vi "Micro-PL Drive Calibration v10.5.1.vi"() -> ()   [LabVIEW 2010]
uses:
  <vilib>/Utility/miscctls.llb/LVPointTypeDef.ctl
  subvi/ESA-C/TypeDefs/ESA-C Connection Settings.ctl
  <vilib>/Utility/file.llb/Write To Spreadsheet File (DBL).vi
panel:
  in  "Snapshot Folder":path=path "C:/Users/WET-KORR/Desktop/Screenshots"
  in  "Camera Name":string="HD USB Camera"
  in  "GPIB-Port":u8=4 max=150 step=1
  in  "Start":bool
  out "Voltages":ext[][](array[numeric])
  out "Current Voltage":ext caption="Current (V)" format="%.1f"
  in  "Axis":u16(ring)=1 items=["X"=1, "Y"=2, "Z"=3]
  out "Progress":u8(slide) max=10 scale=0.0..100.0
  in  "Exit":bool
  in  "Voltage Step":dbl=1.0 caption="Step (V)" min=0.1 max=30.0 step=0.1
  # "Drive Calibration"
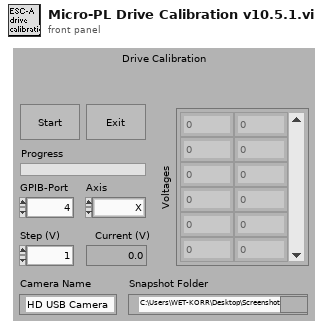
[diagram p1: front panel]
types:
  T1 = typedef "LVPointTypeDef.ctl" = cluster{"Horizontal":i16, "Vertical":i16}
  T2 = typedef "ESA-C Connection Settings.ctl" = cluster{"Objective GPIB-Port":i32, "Stage GPIB-Port":i32, "Drive Selector":u16, "Drive Velocity (V/s)":dbl}
  T3 = typedef "ESA-C Current Values.ctl" = cluster{"Voltages":cluster{"Drive X Voltage":dbl, "Drive Y Voltage":dbl, "Drive Z Voltage":dbl}, "Position":cluster{"Drive X Position":dbl, "Drive Y Position":dbl, "Drive Z Position":dbl}}
  T4 = cluster{"Drive X Voltage":dbl, "Drive Y Voltage":dbl, "Drive Z Voltage":dbl}
  T5 = enum32{"invalid app kind", "Development System", "Run Time System", "Student Edition", "Embedded LabVIEW", "Evaluation", "Custom"}
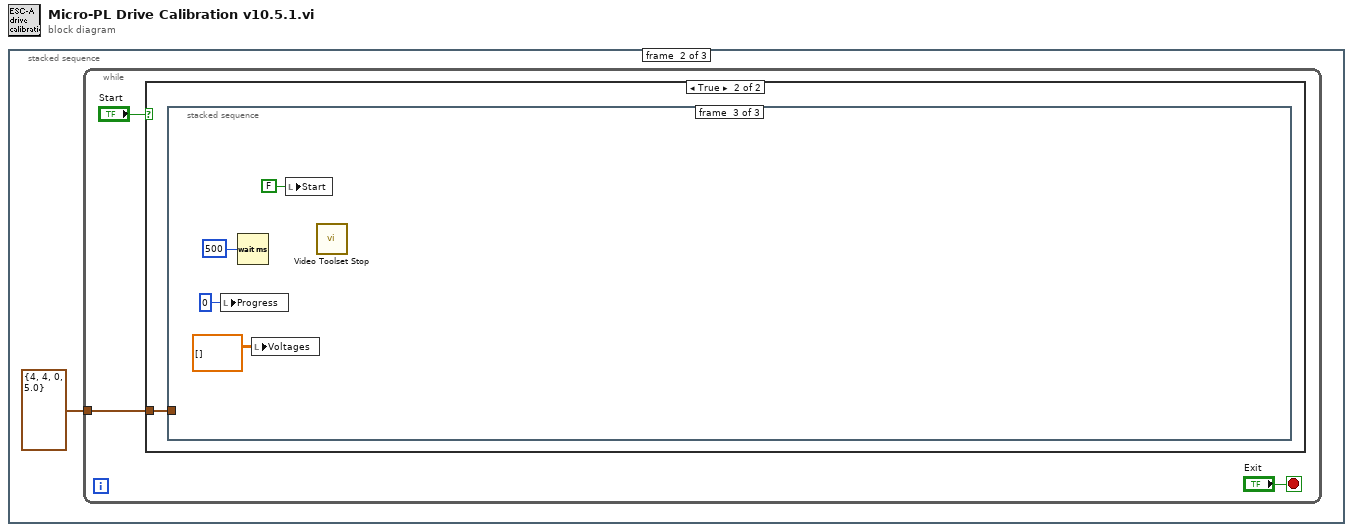
[diagram p0: block diagram]
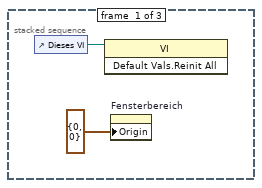
[diagram p2: hidden frame]
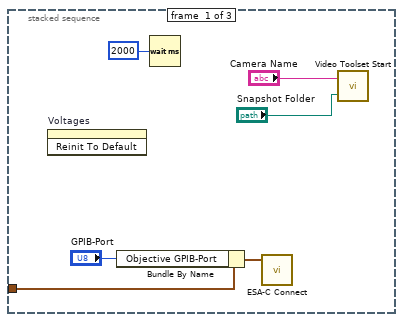
[diagram p4: hidden frame]
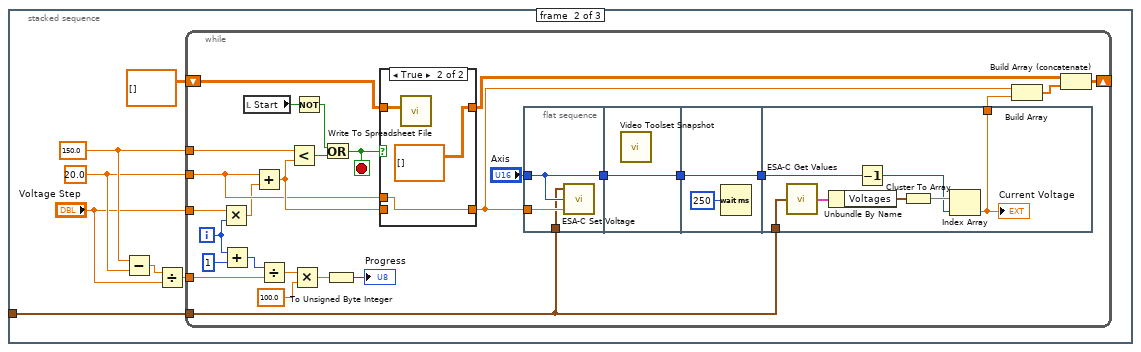
[diagram p5: hidden frame]
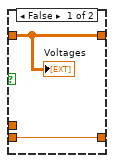
[diagram p6: hidden frame]
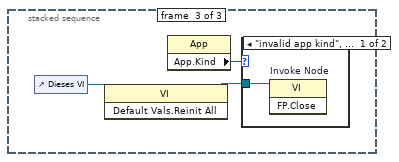
[diagram p7: hidden frame]
diagram:
  n1 = stacked-sequence {
    frame #0 {
      n2 = control-ref of="Dieses VI"() -> (w1:refnum<vi>)
      n3 = invoke class="VI" method="Default Vals.Reinit All"(reference=w1) -> ()  [unwired: 2 in, 3 out]
      n4 = property on="Fensterbereich" class="Pane"("Origin"=T1 {"Horizontal"=0, "Vertical"=0}) -> ()  [unwired: 2 in, 2 out]
    }
    frame #1 {
      n5 = while {
        tunnel: T2 {"Objective GPIB-Port"=4, "Stage GPIB-Port"=4, "Drive Selector"=0, "Drive Velocity (V/s)"=5.0} ("Drive Connection Settings") -> [w4]
        stop <- "Exit" stop-if-true
        n6 = case shown="True" "Start" {
          tunnel: w4 -> [_ w7]
          frame False {
          }
          frame True {
            n7 = stacked-sequence {
              tunnel: w7 -> [w12 w15 _]
              frame #0 {
                n8 = invoke on="Voltages" class="Arr (strikt)" method="Reinit To Default"() -> ()  [unwired: 3 in, 3 out]
                n9 = Bundle By Name(cluster=w12, "Objective GPIB-Port"="GPIB-Port") -> (w11:T2)
                n10 = Wait (ms)(milliseconds to wait=u32 2000 ("Timer-Wert (ms)")) -> ()  [unwired: 1 out]
                n11 = call "ESA-C Connect.vi"("Drive Connection Settings"=w11) -> ()  [unwired: 3 in, 1 out]
                n12 = call "Video Toolset Start.vi"("Snapshot Folder"="Snapshot Folder", "Camera Name"="Camera Name") -> ()  [unwired: 1 in]
              }
              frame #1 {
                w20 = 150.0 ("y")
                w19 = 20.0 ("y")
                n13 = Subtract(x=w20, y=w19) -> (x-y=w18:dbl)
                n14 = Divide(x=w18, y="Voltage Step") -> (x/y=w16:dbl)
                n15 = while {
                  tunnel: w19 -> [w35]
                  tunnel: "Voltage Step" -> [w25]
                  tunnel: w20 -> [w39]
                  tunnel: w16 -> [w41]
                  tunnel: w15 -> [w32]
                  shift-right: [w29] -> _
                  shift-left: dbl[][] [] -> [w28]
                  i -> [w26]
                  stop <- w46 stop-if-true
                  n16 = Multiply(x=w25, y=w26) -> (x*y=w24:dbl)
                  n17 = Add(x=w26, y=1) -> (x+y=w42:i32)
                  n18 = local read "Start"() -> (w37:bool)
                  n19 = Add(x=w35, y=w24) -> (x+y=w38:dbl)
                  n20 = Divide(x=w42, y=w41) -> (x/y=w47:dbl)
                  n21 = Less?(x=w39, y=w38) -> (x < y?=w48:bool)
                  n22 = Multiply(x=w47, y=100.0) -> (x*y=w45:dbl)
                  n23 = Not(x=w37) -> (.not. x?=w36:bool)
                  n24 = Or(x=w36, y=w48) -> (x .or. y?=w46:bool)
                  n25 = To Unsigned Byte Integer(number=w45) -> (unsigned 8bit integer=→"Progress":u8)
                  n26 = case shown="True" w46 {
                    tunnel: w38 -> [w63 _]
                    tunnel: w35 -> [_ w66]
                    tunnel: [w63 w66] -> w23
                    tunnel: w28 -> [w62 w65]
                    tunnel: [w62 dbl[][] []] -> w27
                    frame False {
                      "Voltages" <- w62
                    }
                    frame True {
                      n27 = call-poly <vilib>:"Write To Spreadsheet File.vi"("2D data"=w65) -> ()  [unwired: 7 in, 1 out]
                    }
                  }
                  n28 = flat-sequence {
                    tunnel: w23 -> [w50]
                    tunnel: "Axis" -> [w51]
                    tunnel: [w51] -> w21
                    tunnel: w32 -> [w49]
                    tunnel: w21 -> [w52]
                    tunnel: [w52] -> w22
                    tunnel: [w54] -> w34
                    tunnel: w22 -> [w54]
                    tunnel: w34 -> [w56]
                    tunnel: w32 -> [w61]
                    tunnel: [w58] -> w31
                    frame #0 {
                      n29 = call "ESA-C Set Voltage.vi"("Voltage"=w50, "Axis"=w51, "Drive Connection Settings"=w49) -> ()  [unwired: 2 in]
                    }
                    frame #1 {
                      n30 = call "Video Toolset Snapshot.vi"() -> ()  [unwired: 12 in]
                    }
                    frame #2 {
                      n31 = Wait (ms)(milliseconds to wait=u32 250) -> ()  [unwired: 1 out]
                    }
                    frame #3 {
                      n32 = call "ESA-C Get Values.vi"("Drive Connection Settings"=w61) -> ("Drive Current Values"=w60:T3)
                      n33 = Unbundle By Name(w60) -> ("Voltages"=w59:T4)
                      n34 = Decrement(x=w56) -> (x-1=w55:u16)
                      n35 = Cluster To Array(cluster=w59) -> (array=w57:dbl[])
                      n36 = Index Array(array=w57, index=w55) -> (element=w58:dbl)
                      "Current Voltage" <- w58
                    }
                  }
                  n37 = Build Array(w23, w31) -> (w30:dbl[])
                  n38 = Build Array (concatenate)(w27, w30) -> (w29:dbl[][])
                }
              }
              frame #2 {
                n39 = local write "Progress"(u8 0 ("Progress")) -> ()
                n40 = Wait (ms)(milliseconds to wait=u32 500 ("Timer-Wert (ms)")) -> ()  [unwired: 1 out]
                n41 = local write "Voltages"(ext[][] [] ("Voltages")) -> ()
                n42 = local write "Start"(FALSE ("Start")) -> ()
                n43 = call "Video Toolset Stop.vi"() -> ()  [unwired: 3 in]
              }
            }
          }
        }
      }
    }
    frame #2 {
      n44 = control-ref of="Dieses VI"() -> (w73:refnum<vi>)
      n45 = invoke class="VI" method="Default Vals.Reinit All"(reference=w73) -> (reference out=w71:refnum<vi>)  [unwired: 2 in, 2 out]
      n46 = property class="App"() -> ("App.Kind"=w72:T5)  [unwired: 2 in, 2 out]
      n47 = case shown="\"invalid app kind\", Default" w72 {
        tunnel: w71 -> [w74 _]
        frame "invalid app kind", Default {
          n48 = invoke on="Invoke Node" class="VI" method="FP.Close"(reference=w74) -> ()  [unwired: 2 in, 3 out]
        }
        frame "Development System" {
        }
      }
    }
  }
